vi "Test Apply IMAQdx Attributes from JSON.vi"(11 "Test Case In":refnum<class "Apply IMAQdx Attributes From JSON.lvclass">) -> (0 "error out":errorcluster, 3 "Test Case Out":refnum<class "Apply IMAQdx Attributes From JSON.lvclass">)   [LabVIEW 2024, in "Apply IMAQdx Attributes From JSON.lvclass"]
uses:
  Apply IMAQdx Attributes From JSON.lvclass
  Apply IMAQdx Attributes From JSON.lvclass/Apply IMAQdx Attributes From JSON.ctl
  <vilib>/vision/driver/NI_Vision_Acquisition_Software.lvlib
  <vilib>/userDefined/High Color/IMAQdx.ctl
  Source/Configure Strategies/IMAQdx Strategies/Base/IMAQdx Base Configure Strategy.lvclass
  <vilib>/Astemes/LUnit/Test Case.lvclass
  <vilib>/JDP Science/JSONtext/JSONtext.lvlib
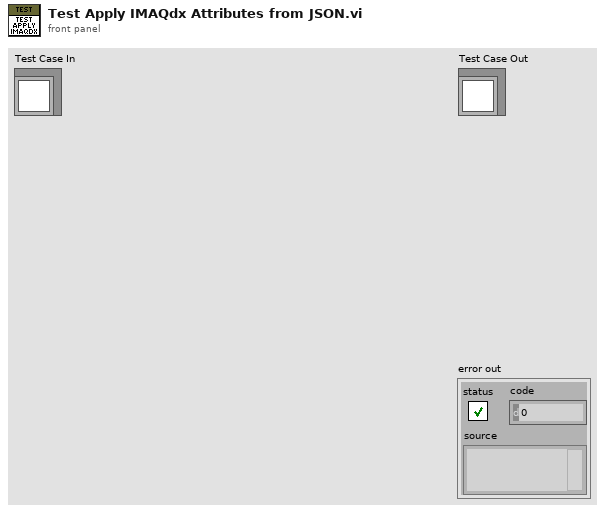
[diagram p1: front panel]
types:
  T1 = typedef "IMAQdx.ctl" = refnum<k21>
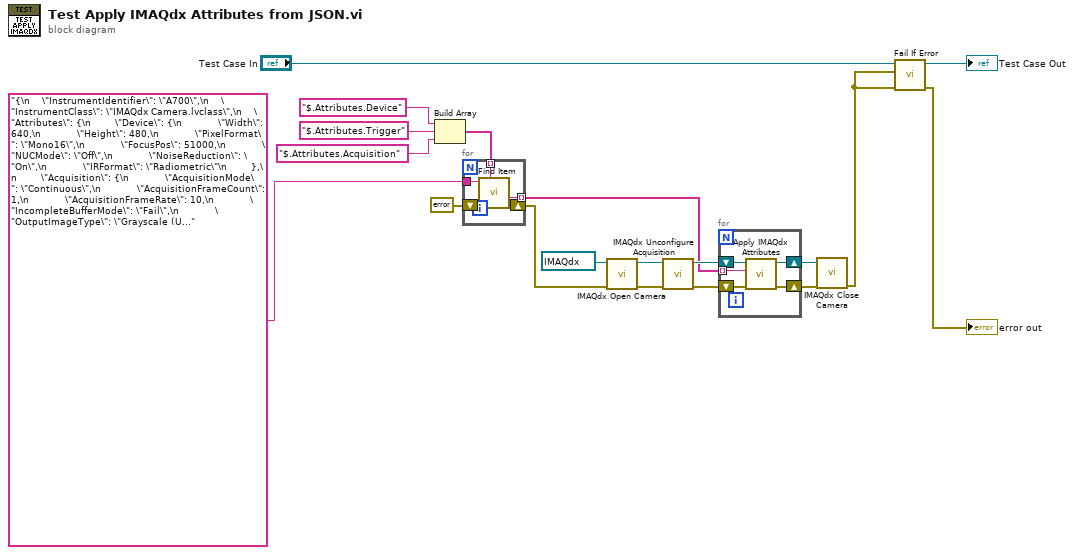
[diagram p0: block diagram]
diagram:
  n1 = Build Array("$.Attributes.Device" ("$Path or Item Name"), "$.Attributes.Trigger" ("$Path or Item Name"), "$.Attributes.Acquisition" ("$Path or Item Name")) -> (w1:string[])
  n2 = for {
    shift-right: [w21] -> w6
    shift-left: errorcluster {"status"=FALSE, "code"=0, "source"=""} ("error out") -> [_]
    tunnel: w1 -> [w20] mode=indexing
    tunnel: "{\n    \"InstrumentIdentifier\": \"A700\",\n    \"InstrumentClass\": \"IMAQdx Camera.lvclass\",\n    \"Attributes\": {\n        \"Device\": {\n            \"Width\": 640,\n            \"Height\": 480,\n            \"PixelFormat\": \"Mono16\",\n            \"FocusPos\": 51000,\n            \"NUCMode\": \"Off\",\n            \"NoiseReduction\": \"On\",\n            \"IRFormat\": \"Radiometric\"\n        },\n        \"Acquisition\": {\n            \"AcquisitionMode\": \"Continuous\",\n            \"AcquisitionFrameCount\": 1,\n            \"AcquisitionFrameRate\": 10,\n            \"IncompleteBufferMode\": \"Fail\",\n            \"OutputImageType\": \"Grayscale (U16)\",\n            \"OverwriteMode\": \"Fail\"\n        },\n        \"Trigger\": {\n            \"TriggerSelector\": \"AcquisitionStart\",\n            \"TriggerMode\": \"On\",\n            \"TriggerSource\": \"Line0\",\n            \"TriggerActivation\": \"RisingEdge\",\n            \"TriggerDelay\": 0\n        }\n    }\n}" -> [w23]
    tunnel: [w22] -> w7 mode=indexing
    n3 = call <vilib>:"Find Item.vi"("$Path or Item Name"=w20, "JSON"=w23) -> ("error out"=w21:errorcluster, "<JSON>"=w22:string)  [unwired: 6 in, 2 out]
  }
  n4 = call <vilib>:"IMAQdx Open Camera.vi"("error in"=w6, "Session In"=T1 "a700") -> ("error out"=w14:errorcluster, "Session Out"=w15:T1)  [unwired: 8 in]
  n5 = call <vilib>:"IMAQdx Unconfigure Acquisition.vi"("error in"=w14, "Session In"=w15) -> ("error out"=w13:errorcluster, "Session Out"=w11:T1)  [unwired: 8 in]
  n6 = for {
    tunnel: w7 -> [w25] mode=indexing
    shift-right: [w27] -> w12
    shift-left: w13 -> [w28]
    shift-right: [w24] -> w5
    shift-left: w11 -> [w26]
    n7 = call "Apply IMAQdx Attributes.vi"("error in"=w28, "<JSON>"=w25, "IMAQdx Session in"=w26) -> ("error out"=w27:errorcluster, "Refnum out"=w24:T1)  [unwired: 7 in]
  }
  n8 = call <vilib>:"IMAQdx Close Camera.vi"("error in"=w12, "Session In"=w5) -> ("error out"=w10:errorcluster)  [unwired: 9 in]
  n9 = call <vilib>:"Fail If Error.vi"("error in (no error)"=w10, "Assert error"=w10, "LUnit Test Case In"="Test Case In") -> ("error out"=→"error out":errorcluster, "LUnit Test Case Out"=→"Test Case Out":refnum<class "Apply IMAQdx Attributes From JSON.lvclass">)  [unwired: 7 in]
